vi "Variant Extract Element.vi"(6 "Dats Start Pos":i32, 9 "data string":string, 10 "Descriptor Pos":i32, 11 "Type Descriptor":i16[](array[numeric])) -> (2 "Data End Pos":i32, 3 "Element":T2)   [LabVIEW 2020, in "Library Commun.lvlib" / "JSON Scalar.lvclass"]
doc: "Extracts an element \"Type Descriptor\" from the compound decriptor array"
uses:
  JSON Scalar.lvclass
  <vilib>/Utility/VariantDataType/Type.ctl
  <vilib>/Utility/VariantDataType/VariantType.lvlib
panel:
  in  "error in":errorcluster
  out "error out":errorcluster
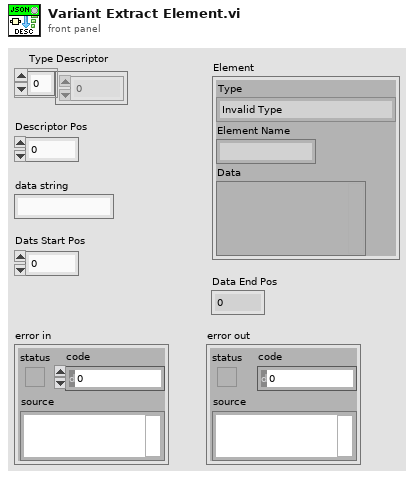
[diagram p1: front panel]
types:
  T1 = typedef "VariantType.lvlib/Type.ctl" = enum8{"Invalid Type", "Void", "I8", "I16", "I32", "I64", "U8", "U16", "U32", "U64", "Single Float", "Double Float", "Extended Float", "Single Complex", "Double Complex", "Extended Complex", "Enum U8", "Enum U16", "Enum U32", "Enum U64", "Single Float With Unit", "Double Float With Unit", "Extended Float With Unit", "Single Complex with Unit", "Double Complex with Unit", "Extended Complex with Unit", "Boolean", "String", "Path", "Picture", "Tag", "Array", "Cluster", "Variant", "LV Variant", "Waveform", "Timestamp", "Digital Waveform", "Digital Data", "ExpressData", "Refnum", "External Data", "VI", "Poly VI", "LabVIEW Class Instance", "Fixed Point"}
  T2 = cluster{"Type":T1, "Element Name":string, "Data":variant}
  T3 = typedef "Library Commun.lvlib/JSON Scalar.lvclass/Variant Data Typdef.ctl" = cluster{"Type Enum":T1, "Name":string, "Variant":variant}
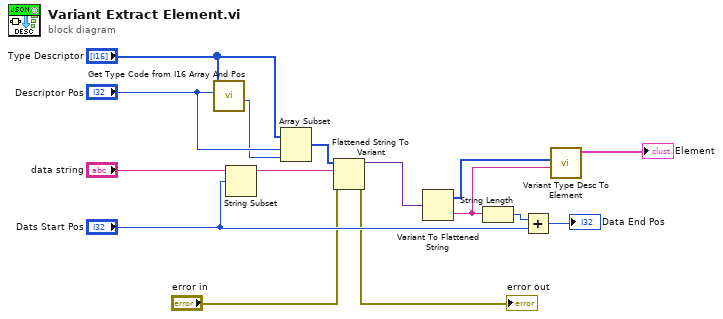
[diagram p0: block diagram]
diagram:
  n1 = call <vilib>:"Get Type Code from I16 Array And Pos.vi"("Pos in Type Descriptor (0)"="Descriptor Pos", "Type descriptor"="Type Descriptor") -> ("Size (Words)"=w7:i32)  [unwired: 7 in, 2 out]
  n2 = String Subset(string="data string", offset (0)="Dats Start Pos") -> (substring=w10:string)  [unwired: 1 in]
  n3 = Array Subset(array="Type Descriptor", index="Descriptor Pos", length=w7) -> (w12:i16[])
  n4 = Flattened String To Variant(4:"error in", 6:w10, 7:w12) -> (0:→"error out":errorcluster, 3:w15:variant)
  n5 = Variant To Flattened String(Variant=w15) -> (data string=w2:string, 1:w3:i16[])
  n6 = String Length(string=w2) -> (length=w8:i32)
  n7 = Add(x=w8, y="Dats Start Pos") -> (x+y=→"Data End Pos":i32)
  n8 = call "Variant Type Desc To Element.vi"("Data String"=w2, "Type Descriptor"=w3) -> ("Variant List"=→"Element":T3)  [unwired: 9 in]
